vi "Mutex Timed Lock (absolute timespec).vi"(8 "error in (no error)":errorcluster, 10 "absolute time (timespec)":cluster{"sec":u64, "nsec":u64}, 11 "Mutex in":T1) -> (0 "error out":errorcluster, 2 "timed out?":bool, 3 "Mutex out":T1)   [LabVIEW 2013, in "Linux RT IPC.lvlib" / "POSIX Threads.lvlib" / "Mutex.lvclass"]
doc: "Calls pthread_mutex_timedlock() on the pthread mutex object encapsulated by Mutex.\n\nThis VI attempts to lock the provided mutex in a specified timeout period. To provide a valid absolute timeout, query the Realtime clock for the current time and offset the time by the desired timeout duration.\n\nRefer to online POSIX documentation for more information."
uses:
  Mutex.lvclass
  Controls/reference.ctl
  POSIX Thread Object/POSIX Thread Object.lvclass/POSIX Thread Object.ctl
  POSIX Thread Object/Private VIs/libpthread path.vi
  <vilib>/NI/NI Linux RT Utilities/VIs/Public/Convert Types/convert timespec 64 to timespec 32.vi
  POSIX Thread Object/Private VIs/get pthread error.vi
  POSIX Thread Object/POSIX Thread Object.lvclass
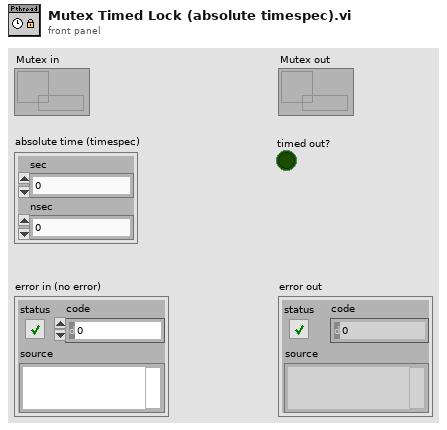
[diagram p1: front panel]
types:
  T1 = typedef "Linux RT IPC.lvlib/POSIX Threads.lvlib/Mutex.lvclass/reference.ctl" = refnum<data-value>
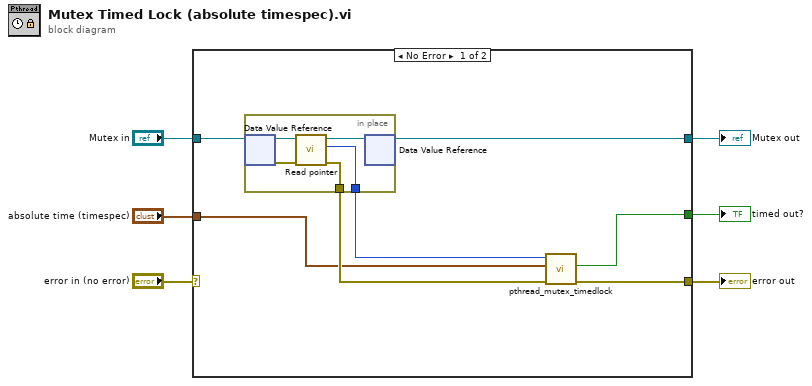
[diagram p0: block diagram]
diagram:
  n1 = case shown="No Error" "error in (no error)" {
    selector: "error in (no error)" -> [_ w20]
    tunnel: [w13 w20] -> w5
    tunnel: "Mutex in" -> [w11 w19]
    tunnel: [w10 w19] -> w3
    tunnel: "absolute time (timespec)" -> [w7 _]
    tunnel: [w12 _] -> w1
    frame No Error {
      n2 = in-place {
        in-place-border: [w15] -> w9
        in-place-border: [w14] -> w8
        n3 = in-place-dvr #1(w11) -> (w18:refnum<class "Mutex.lvclass">, w16:errorcluster)
        n4 = call "Read pointer.vi"("error in (no error)"=w16, "POSIX Thread Object in"=w18) -> ("error out"=w15:errorcluster, "pointer"=w14:u64, "POSIX Thread Object out"=w17:refnum<class "Mutex.lvclass">)  [unwired: 7 in]
        n5 = in-place-dvr #1(w17) -> (w10:T1)  [unwired: 1 out]
      }
      n6 = call "pthread_mutex_timedlock.vi"("error in (no error)"=w9, "absolute time"=w7, "mutex ptr in"=w8) -> ("error out"=w13:errorcluster, "timed out?"=w12:bool)  [unwired: 6 in, 1 out]
    }
    frame Error {
    }
  }
  "Mutex out" <- w3
  "error out" <- w5
  "timed out?" <- w1
